vi "VelocityCommand.vi"(5 "intervalo":dbl=0.016, 6 "MaxOutputXY":dbl=3.0, 7 "estimatives":T1, 8 "Velocities Y":dbl[](array[numeric]), 9 "Time Y":dbl[](array[numeric]), 10 "Velocities X":dbl[](array[numeric]), 11 "Time X":dbl[](array[numeric])) -> (1 "Vy":dbl, 2 "Vx":dbl)   [LabVIEW 2023]
uses:
  Controls/estimatives.ctl
  <vilib>/Analysis/_algsub.llb/Real Vector Norm.vi
  <vilib>/Analysis/NI_AALPro.lvlib
panel:
  out "Velocity Profile Y":cluster{dbl[], dbl[]}[](graph)
  out "Velocity Profile X":cluster{dbl[], dbl[]}[](graph)
  in  "est_vx":dbl
  in  "est_vy":dbl
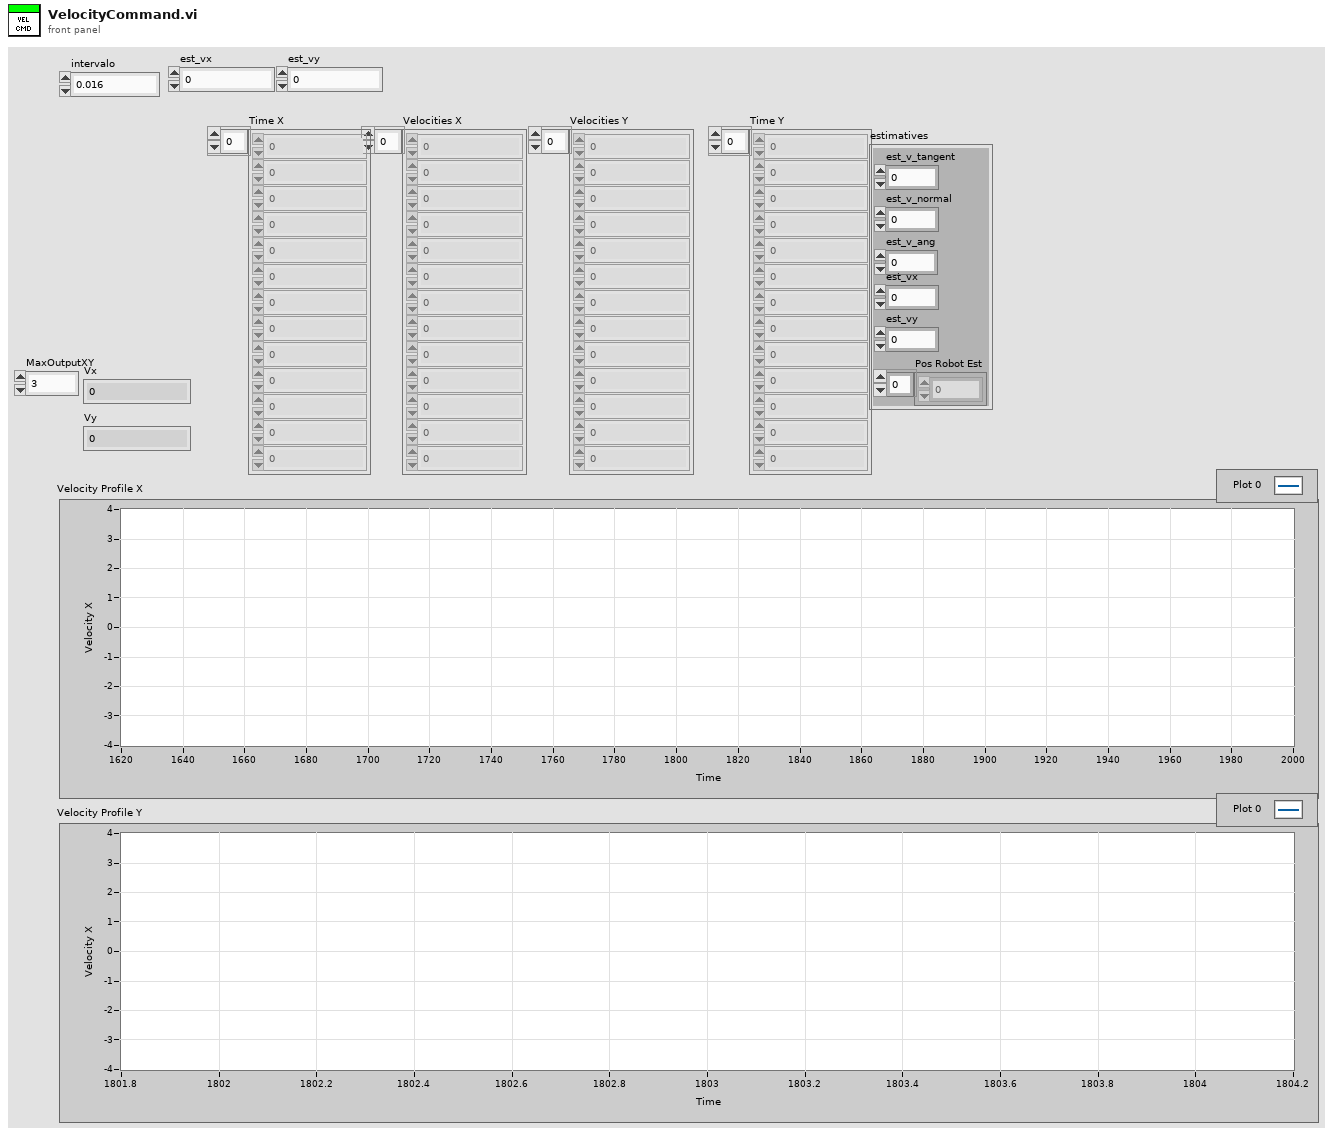
[diagram p1: front panel]
types:
  T1 = typedef "estimatives.ctl" = cluster{"est_v_tangent":dbl, "est_v_normal":dbl, "est_vx":dbl, "est_vy":dbl, "Pos Robot Est":dbl[], "est_v_ang":dbl}
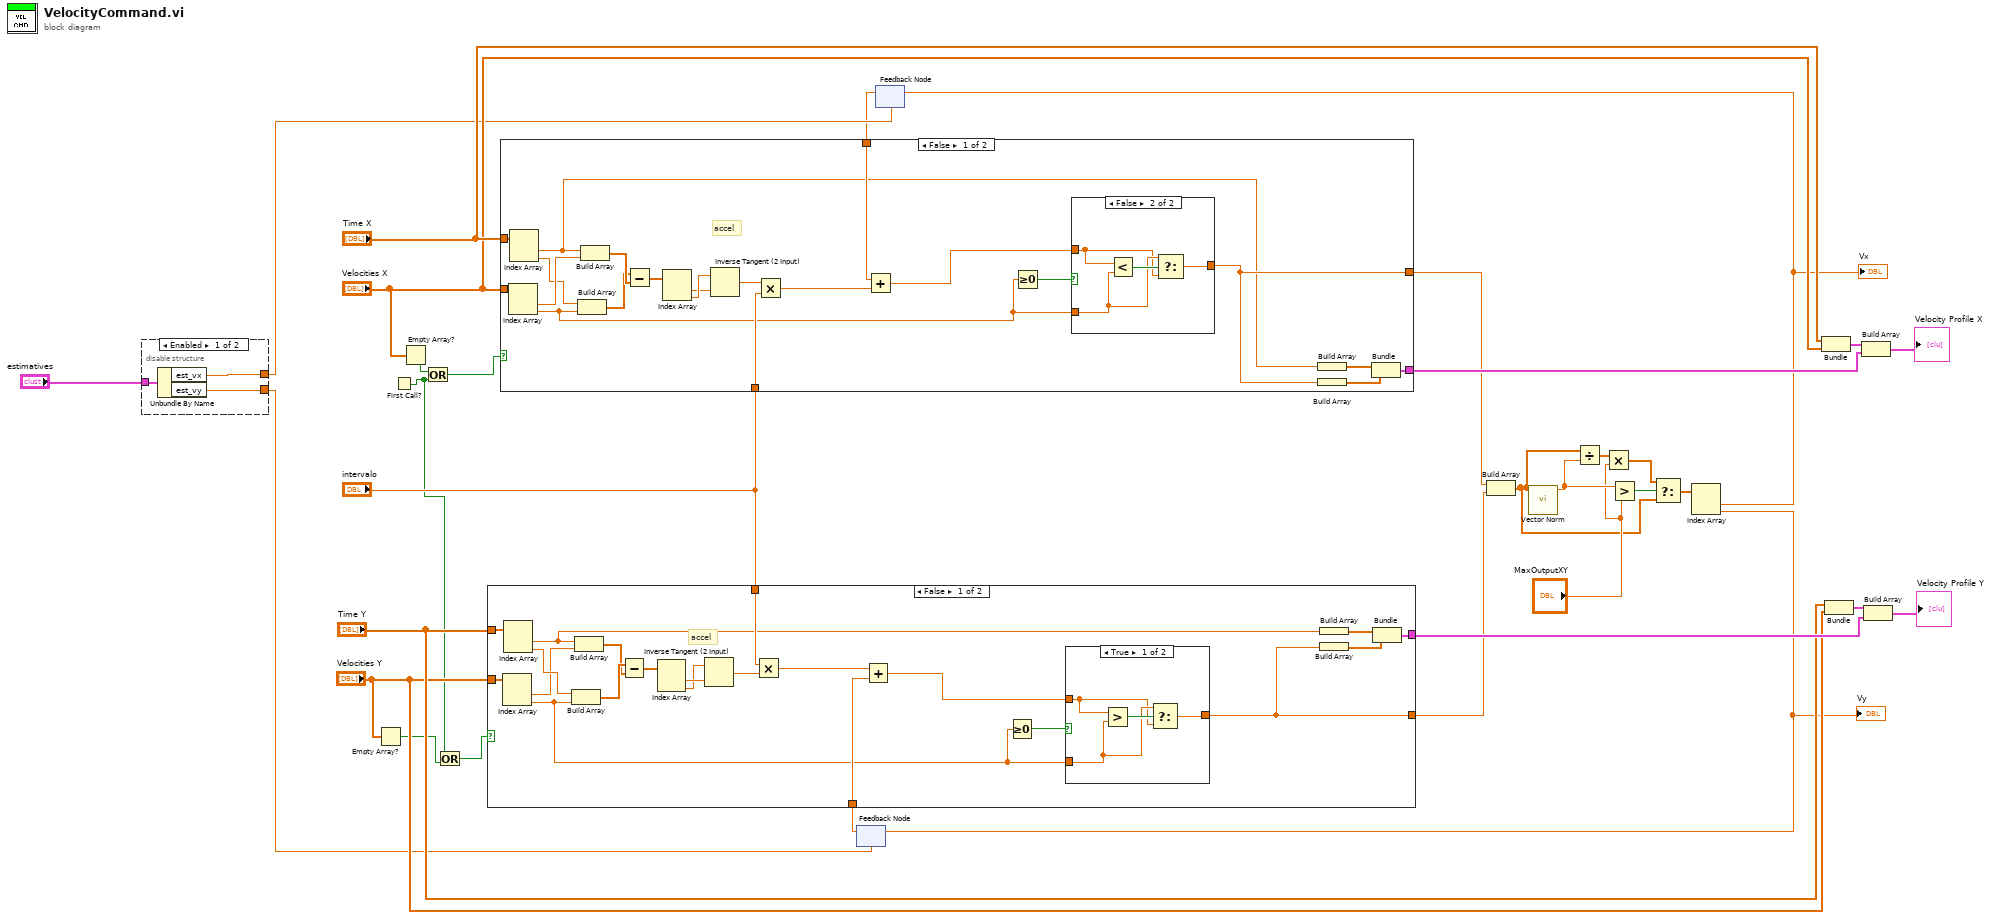
[diagram p0: block diagram]
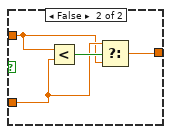
[diagram p2: hidden frame]
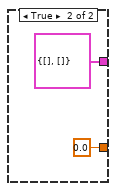
[diagram p3: hidden frame]
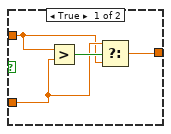
[diagram p4: hidden frame]
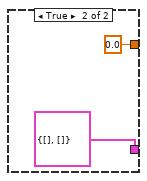
[diagram p5: hidden frame]
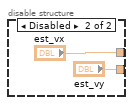
[diagram p6: hidden frame]
diagram:
  n1 = disable-structure shown="Enabled" {
    disable-tunnel: "estimatives" -> [w35 _]
    disable-tunnel: [w34 "est_vx"] -> w16
    disable-tunnel: [w33 "est_vy"] -> w15
    frame Enabled {
      n2 = Unbundle By Name(w35) -> ("est_vx"=w34:dbl, "est_vy"=w33:dbl)
    }
    frame Disabled {
    }
  }
  n3 = Empty Array?(array="Velocities Y") -> (empty?=w19:bool)
  n4 = First Call?() -> (First Call?: T/F=w18:bool)
  n5 = Empty Array?(array="Velocities X") -> (empty?=w21:bool)
  n6 = Or(x=w21, y=w18) -> (x .or. y?=w20:bool)
  n7 = Or(x=w18, y=w19) -> (x .or. y?=w17:bool)
  n8 = feedback #1(w15) -> (w13:dbl)
  n9 = case shown="False" w17 {
    tunnel: "intervalo" -> [w58 _]
    tunnel: [w57 cluster{dbl[], dbl[]} {[], []}] -> w27
    tunnel: "Velocities Y" -> [w56 _]
    tunnel: "Time Y" -> [w55 _]
    tunnel: w13 -> [w54 _]
    tunnel: [w53 0.0 ("v3")] -> w11
    frame False {
      # "accel"
      n10 = Index Array(array=w56) -> (element #1=w46:dbl, element #2=w41:dbl)  [unwired: 2 in]
      n11 = Index Array(array=w55) -> (element #1=w38:dbl, element #2=w47:dbl)  [unwired: 2 in]
      n12 = Build Array(w47, w41) -> (w49:dbl[])
      n13 = Build Array(w38, w46) -> (w48:dbl[])
      n14 = Subtract(x=w49, y=w48) -> (x-y=w50:dbl[])
      n15 = Index Array(array=w50) -> (element #1=w52:dbl, element #2=w51:dbl)  [unwired: 2 in]
      n16 = Inverse Tangent (2 Input)(1:w52, 2:w51) -> (0:w45:dbl)
      n17 = Multiply(x=w58, y=w45) -> (x*y=w44:dbl)
      n18 = Add(x=w44, y=w54) -> (x+y=w42:dbl)
      n19 = Greater Or Equal To 0?(x=w41) -> (x >= 0?=w43:bool)
      n20 = case shown="True" w43 {
        tunnel: w42 -> [w60 w64]
        tunnel: w41 -> [w61 w65]
        tunnel: [w59 w63] -> w53
        frame True {
          n21 = Greater?(x=w60, y=w61) -> (0:w62:bool)
          n22 = Select(t=w61, s=w62, f=w60) -> (s? t:f=w59:dbl)
        }
        frame False {
          n23 = Less?(x=w64, y=w65) -> (x < y?=w66:bool)
          n24 = Select(t=w65, s=w66, f=w64) -> (s? t:f=w63:dbl)
        }
      }
      n25 = Build Array(w38) -> (w40:dbl[])
      n26 = Build Array(w53) -> (w39:dbl[])
      n27 = Bundle(w40, w39) -> (w57:cluster{dbl[], dbl[]})  [unwired: 1 in]
    }
    frame True {
    }
  }
  n28 = feedback #2(w16) -> (w14:dbl)
  n29 = case shown="False" w20 {
    tunnel: "intervalo" -> [w89 _]
    tunnel: [w88 cluster{dbl[], dbl[]} {[], []} ("Cluster")] -> w29
    tunnel: "Time X" -> [w87 _]
    tunnel: w14 -> [w86 _]
    tunnel: [w85 0.0 ("v3")] -> w12
    tunnel: "Velocities X" -> [w84 _]
    frame False {
      # "accel"
      n30 = Index Array(array=w84) -> (element #1=w83:dbl, element #2=w72:dbl)  [unwired: 2 in]
      n31 = Index Array(array=w87) -> (element #1=w69:dbl, element #2=w82:dbl)  [unwired: 2 in]
      n32 = Build Array(w82, w72) -> (w80:dbl[])
      n33 = Build Array(w69, w83) -> (w81:dbl[])
      n34 = Subtract(x=w80, y=w81) -> (x-y=w79:dbl[])
      n35 = Index Array(array=w79) -> (element #1=w77:dbl, element #2=w78:dbl)  [unwired: 2 in]
      n36 = Inverse Tangent (2 Input)(1:w77, 2:w78) -> (0:w76:dbl)
      n37 = Multiply(x=w76, y=w89) -> (x*y=w75:dbl)
      n38 = Add(x=w86, y=w75) -> (x+y=w73:dbl)
      n39 = Greater Or Equal To 0?(x=w72) -> (x >= 0?=w74:bool)
      n40 = case shown="False" w74 {
        tunnel: w73 -> [w91 w95]
        tunnel: w72 -> [w92 w96]
        tunnel: [w90 w94] -> w85
        frame True {
          n41 = Greater?(x=w91, y=w92) -> (0:w93:bool)
          n42 = Select(t=w92, s=w93, f=w91) -> (s? t:f=w90:dbl)
        }
        frame False {
          n43 = Less?(x=w95, y=w96) -> (x < y?=w97:bool)
          n44 = Select(t=w96, s=w97, f=w95) -> (s? t:f=w94:dbl)
        }
      }
      n45 = Build Array(w69) -> (w70:dbl[])
      n46 = Build Array(w85) -> (w71:dbl[])
      n47 = Bundle(w70, w71) -> (w88:cluster{dbl[], dbl[]})  [unwired: 1 in]
    }
    frame True {
    }
  }
  n48 = Build Array(w12, w11) -> (w5:dbl[])
  n49 = call-poly <vilib>:"Vector Norm.vi"("Input Vector"=w5) -> ("norm"=w9:dbl)  [unwired: 9 in, 1 out]
  n50 = Divide(x=w5, y=w9) -> (x/y=w8:dbl[])
  n51 = Multiply(x=w8, y="MaxOutputXY") -> (x*y=w7:dbl[])
  n52 = Greater?(x=w9, y="MaxOutputXY") -> (0:w10:bool)
  n53 = Select(t=w7, s=w10, f=w5) -> (s? t:f=w4:dbl[])
  n54 = Index Array(array=w4) -> (element #1=w3:dbl, element #2=w2:dbl)  [unwired: 2 in]
  "Vx" <- w3
  "Vy" <- w2
  n55 = feedback-in #1(w2) -> ()
  n56 = feedback-in #2(w3) -> ()
  n57 = Bundle("Time X"="Time X", "Velocities X"="Velocities X") -> (w31:cluster{"Time X":dbl[], "Velocities X":dbl[]})  [unwired: 1 in]
  n58 = Bundle("Time Y"="Time Y", "Velocities Y"="Velocities Y") -> (w25:cluster{"Time Y":dbl[], "Velocities Y":dbl[]})  [unwired: 1 in]
  n59 = Build Array(w31, w29) -> (→"Velocity Profile X":cluster{"Time X":dbl[], "Velocities X":dbl[]}[])
  n60 = Build Array(w25, w27) -> (→"Velocity Profile Y":cluster{"Time Y":dbl[], "Velocities Y":dbl[]}[])
